vi "ROIdetection.vi"(8 "Threshold":dbl=100.0, 9 "ROI rect":cluster{i32, i32, i32, i32}, 10 "Img Dst":cluster{"IMAQ ROI":T1, "error in ":errorcluster}, 11 "Image In":T1) -> (0 "condition":bool=TRUE, 1 "StDev bar":dbl(slide)=26.100881576538086 scale=20.0..35.0, 2 "StDev num":sgl, 3 "Image Out":T1)   [LabVIEW 2016]
uses:
  <vilib>/vision/Image Controls.llb/IMAQ Image.ctl
  <vilib>/vision/NI_Vision_Development_Module.lvlib
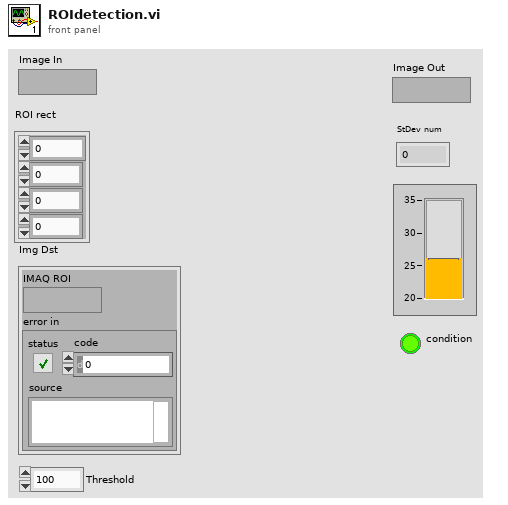
[diagram p1: front panel]
types:
  T1 = typedef "IMAQ Image.ctl" = refnum<image>
  T2 = cluster{"histogram":u32[], "Minimal Value":sgl, "Maximal Value":sgl, "Starting Value":sgl, "Interval Width":sgl, "Mean Value":sgl, "Standard  Variation":sgl, "Area (pixels)":i32}
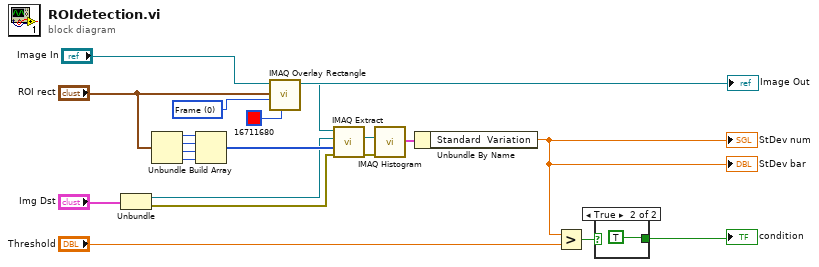
[diagram p0: block diagram]
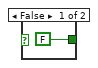
[diagram p2: hidden frame]
diagram:
  w20 = u32 0 items=["Frame", "Fill", "Highlight"] ("Drawing Mode (Frame)")
  n1 = Unbundle("Img Dst") -> ("IMAQ ROI"=w5:T1, "error in"=w4:errorcluster)
  n2 = Unbundle("ROI rect") -> (w10:i32, w9:i32, w8:i32, w7:i32)
  n3 = Build Array(w10, w9, w8, w7) -> (w19:i32[])
  n4 = call "IMAQ Overlay Rectangle"("Color"=u32 16711680, "Drawing Mode (Frame)"=w20, "Rectangle"="ROI rect", "Image"="Image In") -> ("Image Out"=→"Image Out":T1)  [unwired: 6 in, 1 out]
  n5 = call "IMAQ Extract"("Optional Rectangle"=w19, "error in (no error)"=w4, "Image Dst"=w5, "Image Src"="Image In") -> ("error out"=w17:errorcluster, "Image Dst Out"=w16:T1)  [unwired: 6 in]
  n6 = call "IMAQ Histogram"("error in (no error)"=w17, "Image"=w16) -> ("Histogram Report"=w18:T2)  [unwired: 8 in, 1 out]
  n7 = Unbundle By Name(w18) -> ("Standard  Variation"=w14:sgl)
  "StDev num" <- w14
  "StDev bar" <- w14
  n8 = Greater?(x=w14, y="Threshold") -> (0:w13:bool)
  n9 = case shown="True" w13 {
    tunnel: [FALSE ("Worm\ndetected") TRUE ("Worm detected")] -> w11
    frame False {
    }
    frame True {
    }
  }
  "condition" <- w11
